vi "Fit_Poly2Disc.vi"(9 "stopping criteria":T1={"function tolerance"=0.001, "parameter tolerance"=0.001, "max iterations"=100, "max function calls"=1000, "gradient tolerance"=0.001, "max time (sec)"=-1.0}, 10 "Rc":dbl[](array[numeric]), 11 "Xd(t,r)":dbl[][](array[numeric])) -> (0 "f(minimum)":dbl, 1 "Iterations":i32, 2 "Sine Phase":dbl)   [LabVIEW 2022 SP3]
uses:
  <vilib>/gmath/NumericalOptimization/stopping criteria.ctl
  Displacement Data.ctl
  <vilib>/Utility/error.llb/DialogType.ctl
  <vilib>/gmath/NumericalOptimization/Downhill Simplex.vi
  <vilib>/gmath/NI_Gmath.lvlib
panel:
  in  "Display Graph?":bool
  out "XY Graph":cluster{"Rc":dbl[], "Xd(t,r)":dbl[]}[](graph)
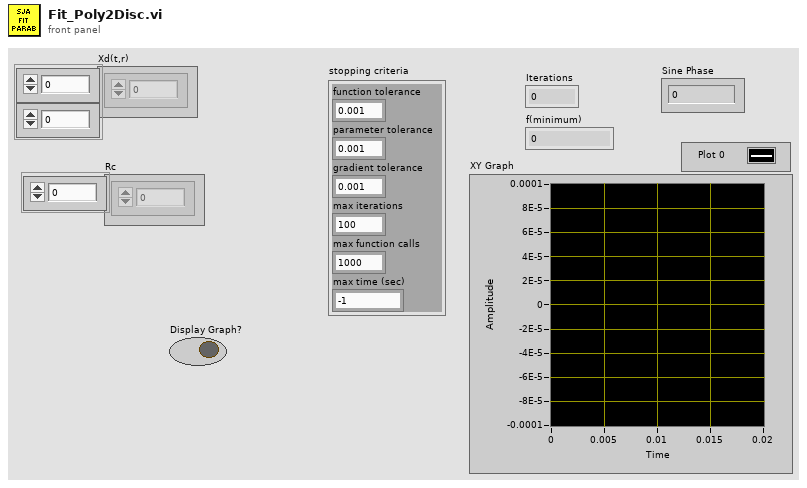
[diagram p1: front panel]
types:
  T1 = typedef "NI_Gmath.lvlib/stopping criteria.ctl" = cluster{"function tolerance":dbl, "parameter tolerance":dbl, "max iterations":i32, "max function calls":i32, "gradient tolerance":dbl, "max time (sec)":dbl}
  T2 = typedef "DialogType.ctl" = u16
  T3 = typedef "Displacement Data.ctl" = cluster{"Xd(t,r)":dbl[][], "Rc":dbl[]}
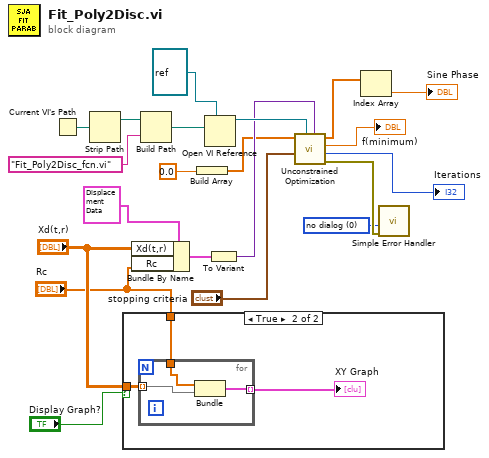
[diagram p0: block diagram]
diagram:
  w1 = T2 0 items=["no dialog", "OK message", "continue or stop message", "OK message + warnings", "continue/stop + warnings"] ("type of dialog (OK msg:1)")
  n1 = Current VI's Path() -> (path=w16:path)
  n2 = Strip Path(path=w16) -> (stripped path=w15:path)  [unwired: 1 out]
  n3 = case shown="True" "Display Graph?" {
    tunnel: "Xd(t,r)" -> [_ w24]
    tunnel: "Rc" -> [_ w23]
    frame False {
    }
    frame True {
      n4 = for {
        tunnel: w24 -> [w27] mode=indexing
        tunnel: w23 -> [w26]
        tunnel: [w25] -> w22 mode=indexing
        n5 = Bundle("Rc"=w26, "Xd(t,r)"=w27) -> (w25:cluster{"Rc":dbl[], "Xd(t,r)":dbl[]})  [unwired: 1 in]
      }
      "XY Graph" <- w22
    }
  }
  n6 = Bundle By Name(cluster=T3 {"Xd(t,r)"=array25x40[1000 elements], "Rc"=[-10.5, -9.5, -8.5, -7.5, -6.5, -5.5, -4.5, -3.5, -2.5, -1.5, -19.5, -0.5, 0.5, 1.5, 2.5, 3.5, 4.5, 5.5, 6.5, 7.5, 8.5, -18.5, 9.5, 10.5, 11.5, 12.5, 13.5, 14.5, 15.5, 16.5, 17.5, 18.5, -17.5, 19.5, -16.5, -15.5, -14.5, -13.5, -12.5, -11.5]} ("Displacement Data"), "Xd(t,r)"="Xd(t,r)", "Rc"="Rc") -> (w11:T3)
  n7 = Build Path(base path=w15, name or relative path="Fit_Poly2Disc_fcn.vi") -> (appended path=w13:path)
  n8 = Build Array(0.0 ("Numeric")) -> (w7:dbl[])
  n9 = Open VI Reference(type specifier VI Refnum (for type only)=refnum<vi> refnum, vi path=w13) -> (vi reference=w20:refnum<vi>)  [unwired: 4 in, 1 out]
  n10 = To Variant(anything=w11) -> (Variant=w17:variant)
  n11 = call-poly <vilib>:"Unconstrained Optimization.vi"("function data"=w17, "objective function"=w20, "stopping criteria"="stopping criteria", "start"=w7) -> ("error out"=w2:errorcluster, "number of function evaluations"=→"Iterations":i32, "f(minimum)"=→"f(minimum)":dbl, "minimum"=w10:dbl[])  [unwired: 4 in]
  n12 = Index Array(array=w10) -> (element=→"Sine Phase":dbl)  [unwired: 1 in]
  n13 = call <vilib>:"Simple Error Handler.vi"("type of dialog (OK msg:1)"=w1, "error in (no error)"=w2) -> ()  [unwired: 3 in, 5 out]
